vi "Is Cell Valid.vi"(9 "y":i32, 10 "x":i32, 11 "cost in":dbl[][](array[numeric])) -> (2 "Valid":bool, 3 "cost out":dbl[][](array[numeric]))   [LabVIEW 2013]
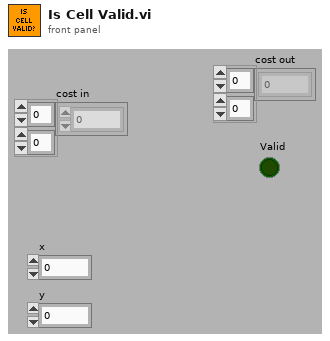
[diagram p1: front panel]
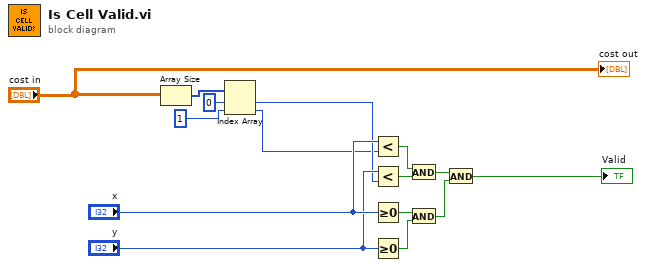
[diagram p0: block diagram]
diagram:
  n1 = Array Size(array="cost in") -> (size(s)=w6:i32[])
  n2 = Index Array(array=w6, index #1=0 ("index"), index #2=1 ("index")) -> (element #1=w3:i32, element #2=w2:i32)
  n3 = Less?(x="x", y=w2) -> (x < y?=w9:bool)
  n4 = Less?(x="y", y=w3) -> (x < y?=w12:bool)
  n5 = Greater Or Equal To 0?(x="x") -> (x >= 0?=w11:bool)
  n6 = Greater Or Equal To 0?(x="y") -> (x >= 0?=w10:bool)
  n7 = And(x=w9, y=w12) -> (x .and. y?=w8:bool)
  n8 = And(x=w11, y=w10) -> (x .and. y?=w7:bool)
  n9 = And(x=w8, y=w7) -> (x .and. y?=→"Valid":bool)
  "cost out" <- "cost in"
